vi "ttm_twocreep_poller.vi"   [LabVIEW 2011]
uses:
  protocols/protocol_TwoCreep/Protocol_TwoCreep.lvclass
types:
  T1 = cluster{"Axis Information":cluster{"Device ID":i32, "Device Name":string, "Device Type":i32}[], "Axis Selector":i32[], "Control Modes out":u16[], "error out":errorcluster, "Channel Data":cluster{"Name":string, "Type":i32, "SI Full Scale":dbl, "Full Scale":dbl, "Units String":string, "Display Format":string, "Gauge Length":dbl}[][]}
  T2 = cluster{"Name":string, "Type":i32, "SI Full Scale":dbl, "Full Scale":dbl, "Units String":string, "Display Format":string, "Gauge Length":dbl}[][]
  T3 = cluster{"Device ID":i32, "Device Name":string, "Device Type":i32}[]
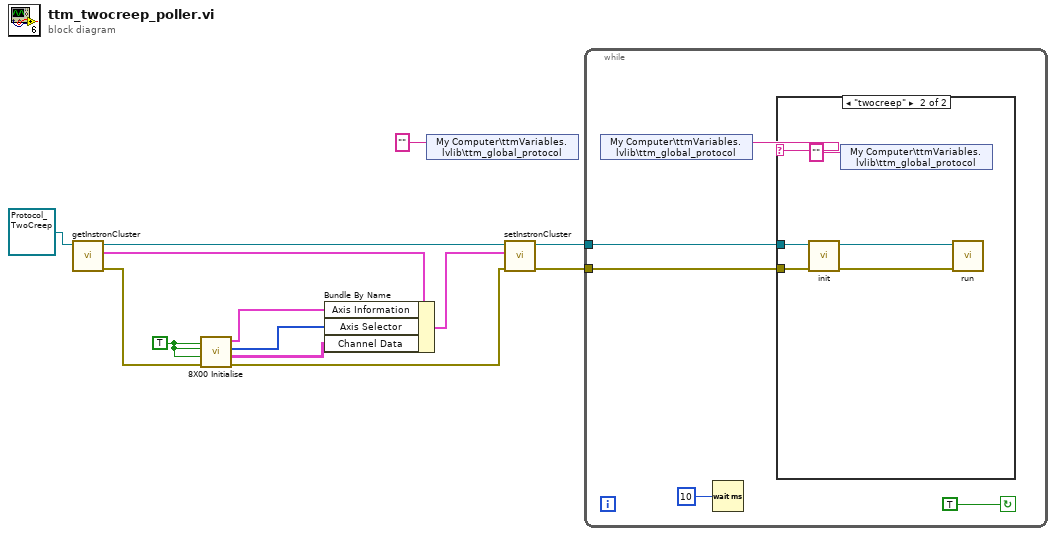
[diagram p0: block diagram]
diagram:
  w12 = TRUE ("Create Console? (T)")
  n1 = call-dynamic "getInstronCluster.vi"("Protocol_Generic in"=refnum<class "Protocol_TwoCreep.lvclass"> refnum ("Protocol_TwoCreep.lvclass")) -> ("error out"=w7:errorcluster, "InstronCluster"=w11:T1, "Protocol_Generic out"=w5:refnum<class "Protocol_TwoCreep.lvclass">)  [unwired: 8 in]
  n2 = call "8X00 Initialise.vi"("error in (no error)"=w7, "Reset?"=w12, "Create DVM? (T)"=w12, "Create Console? (T)"=w12) -> ("error out"=w2:errorcluster, "Channel Data"=w8:T2, "Axis Selector"=w9:i32[], "Axis Information"=w10:T3)
  n3 = Bundle By Name(cluster=w11, "Axis Information"=w10, "Axis Selector"=w9, "Channel Data"=w8) -> (w3:T1)
  n4 = shared-variable "My Computer\\ttmVariables.lvlib\\ttm_global_protocol"("" ("protocol")) -> ()  [unwired: 1 in, 1 out]
  n5 = call-dynamic "setInstronCluster.vi"("error in (no error)"=w2, "InstronCluster"=w3, "Protocol_Generic in"=w5) -> ("error out"=w1:errorcluster, "Protocol_Generic out"=w4:refnum<class "Protocol_TwoCreep.lvclass">)  [unwired: 7 in]
  n6 = while {
    tunnel: w4 -> [w15]
    tunnel: w1 -> [w14]
    stop <- TRUE continue-if-true
    n7 = shared-variable "My Computer\\ttmVariables.lvlib\\ttm_global_protocol"() -> (w16:string)  [unwired: 1 in, 1 out]
    n8 = Wait (ms)(milliseconds to wait=u32 10) -> ()  [unwired: 1 out]
    n9 = case shown="\"twocreep\"" w16 {
      tunnel: w15 -> [_ w22]
      tunnel: w14 -> [_ w19]
      frame "", Default {
      }
      frame "twocreep" {
        n10 = call-dynamic "init.vi"("error in (no error)"=w19, "Protocol_TwoCreep in"=w22) -> ("error out"=w20:errorcluster, "Protocol_TwoCreep out"=w21:refnum<class "Protocol_TwoCreep.lvclass">)  [unwired: 8 in]
        n11 = shared-variable "My Computer\\ttmVariables.lvlib\\ttm_global_protocol"("" ("protocol")) -> ()  [unwired: 1 in, 1 out]
        n12 = call-dynamic "run.vi"("error in (no error)"=w20, "Protocol_TwoCreep in"=w21) -> ()  [unwired: 8 in, 2 out]
      }
    }
  }
